vi "SavedSettingsFilterDummy.vi"(8 "error in (no error)":errorcluster, 9 "Dummy prefix":string="???? ", 10 "Saved Values":map{string, string}(c390), 11 "Control Tree in":refnum<vi>) -> (0 "error out":errorcluster, 1 "Items Found":cluster{string, string}[](array[cluster]), 2 "Items Not Found":string[](array[string]), 3 "Control Tree out":refnum<vi>)   [LabVIEW 2019]
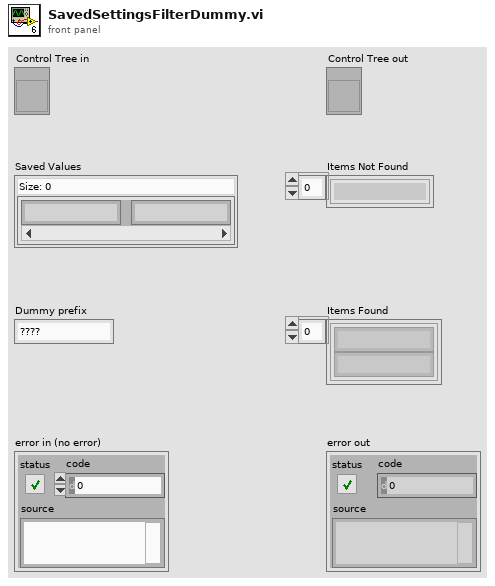
[diagram p1: front panel]
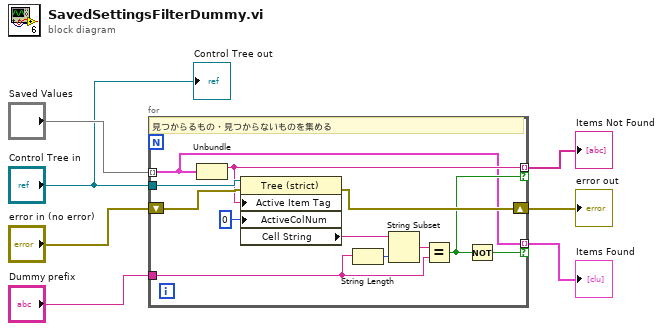
[diagram p0: block diagram]
diagram:
  n1 = for {
    tunnel: "Saved Values" -> [w8] mode=indexing
    tunnel: [w10] -> w4 mode=indexing if=w11
    tunnel: "Control Tree in" -> [w19]
    tunnel: "Dummy prefix" -> [w14]
    shift-right: [w12] -> w7
    shift-left: "error in (no error)" -> [w13]
    tunnel: [w8] -> w1 mode=indexing if=w9
    # "見つからるもの・見つからないものを集める"
    n2 = Unbundle(w8) -> (w10:string)  [unwired: 1 out]
    n3 = property class="Tree (strict)"(reference=w19, error in=w13, "Active Item Tag"=w10, "ActiveColNum"=0 ("Active Cell:Active Column Number")) -> (error out=w12:errorcluster, "Cell String"=w17:string)  [unwired: 1 out]
    n4 = String Length(string=w14) -> (length=w16:i32)
    n5 = String Subset(string=w17, length (rest)=w16) -> (substring=w15:string)  [unwired: 1 in]
    n6 = Equal?(x=w15, y=w14) -> (x = y?=w11:bool)
    n7 = Not(x=w11) -> (.not. x?=w9:bool)
  }
  "error out" <- w7
  "Items Not Found" <- w4
  "Items Found" <- w1
  "Control Tree out" <- "Control Tree in"
